vi "RT_cRIO_AIChar_v3.vi"() -> ()   [LabVIEW 2019]
uses:
  FPGA/TypeDefs/AO mode TabCtrl.ctl
  FPGA/TypeDefs/AI_channelEnum.ctl
  FPGA/TypeDefs/SamplingModeEnum.ctl
  <vilib>/NI/STM/SubVIs/MetaDataElement.ctl
  <vilib>/Platform/TimedLoop/XDataNode/timing_clust.ctl
  <vilib>/Platform/TimedLoop/XDataNode/nitl_modes.ctl
  <vilib>/Platform/TimedLoop/XDataNode/wakeup.ctl
  <vilib>/rvi/Analysis/host/Butterworth/config/Butterworth Filter Order.ctl
  <vilib>/rvi/Analysis/host/Butterworth/config/Butterworth Filter Type.ctl
  <vilib>/NI/STM/TCP/Write Meta Data (TCP Ref).vi
  <vilib>/NI/STM/TCP/Get Connection Reference (TCP).vi
  <vilib>/NI/STM/TCP/Write Meta Data (TCP Clst).vi
  <vilib>/FPGAPlugInAG/cRIO-9064/niLvFpga_Open_cRIO-9064.vi
  <vilib>/rvi/interface/common/dynamic/niFpgaDynamicAddResources.vi
  <vilib>/NI/STM/TCP/Write Message (TCP).vi
  <vilib>/rvi/Analysis/host/Private/Sample Rate To Loop Time (ticks).vi
  <vilib>/rvi/Analysis/host/Butterworth/config/BwScaledCoefficients.vi
  <vilib>/Utility/error.llb/Error Cluster From Error Code.vi
  <vilib>/rvi/errors/niLvFpgaAdjustHostInterfaceError.vi
  <vilib>/FPGAPlugInAG/Dynamic/niLvFpga_Close_Dynamic.vi
  <vilib>/rvi/interface/nirviOpenFPGA/nirviOpenFPGA.xnode
  FPGA Bitfiles/ainoisecharacter_FPGATarget2_FPGAcRIOMainv4_BvJefVyibFQ.lvbitx
  <vilib>/rvi/Analysis/host/Butterworth/XNode/ButterworthCoefficients.xnode
  <vilib>/rvi/interface/nirviReadWriteControl/nirviReadWriteControl.xnode
  <vilib>/Platform/TimedLoop/XDataNode/XDataNode.xnode
  <vilib>/rvi/interface/nirviCloseFPGA/nirviCloseFPGA.xnode
  <vilib>/Platform/TimedLoop/XDataNode/XDNodeRunTimeDep.lvlib
  Components/Timing/Timing.lvlib
  <vilib>/NI/STM/NI STM.lvlib
  <vilib>/rvi/interface/Simulation/niFpgaSimulationCallBeginRW.vi
  NiFpgaLv.dll
  <vilib>/rvi/Analysis/host/Public/NI_FpgaMspHost.lvlib
panel:
  in  "Sampling Mode":T1
  out "AI Process Freq.\ntoo high?":bool
  in  "AI Process Freq. [Hz]":dbl=20000.0 format="%#.3p"
  in  "Select Channel":T2=enum."AI1"
  in  "AO mode":T3=enum."100*AI"
  in  "AO Out [V]":fxp<+/-,18,5>
  in  "AI-chain LPF [Hz]":dbl=500.0 format="%#_6p"
  out "Sample Freq.\ntoo high?":bool
  in  "AO enable?":bool
  in  "Sample Freq [Hz]":dbl=300000.0 format="%#.3p"
  out "RT Loop Rate":dbl=5000.0 format="%.3p"
  out "# of iterations\n[STM write]":i32
  out "# elements \nFIFO buffer":u32
  out "Finished \nlate counter?":dbl
  in  "stop":bool
  # "- Open PC_SensorChar vi and run that VI as well to start capturing data!\n- Sampling Mode : \n     - LPF adds a  butterworth filter after the ADC conversion.\n     - 4pt. Avg adds a 4pt. Moving Avg before the LPF and after ADC."
  # "AO = \n100 * (AI value)"
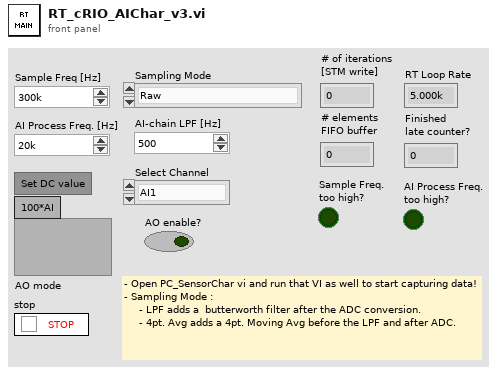
[diagram p1: front panel]
types:
  T1 = typedef "SamplingModeEnum.ctl" = enum16{"Raw", "M64 (ReSpl)", "M128 (ReSpl)", "M256 (ReSpl)", "MA (AI)", "4pt MA (AI) + M64 (ReSpl)", "LPF (Proc.)", "4pt MA (AI) + LPF (Proc.)", "4pt MA (Proc.) + LPF (Proc.)"}
  T2 = typedef "AI_channelEnum.ctl" = enum16{"AI0", "AI1", "AI2", "AI3"}
  T3 = typedef "AO mode TabCtrl.ctl" = enum32{"Set DC value", "100*AI"}
  T4 = typedef "NI STM.lvlib/MetaDataElement.ctl" = string
  T5 = typedef "NI STM.lvlib/TCP Connection Info.ctl" = cluster{"connection ID":refnum<k5>, "meta data":T4[]}
  T6 = typedef "XDNodeRunTimeDep.lvlib/timing_clust.ctl" = cluster{"Expected End [f-1]":u64, "Actual End [f-1]":u64, "Finished Late? [f-1]":bool, "Expected End [i-1]":u64, "Actual End [i-1]":u64, "Finished Late? [i-1]":bool, "Expected Start [i]":u64, "Actual Start [i]":u64, "Expected Start [f]":u64, "Actual Start [f]":u64, "Source Name":string, "Structure Name":string, "Period":i64, "Deadline":i64, "Offset":i64, "Start":i64, "Priority":i32, "Timeout":i32, "Mode":T7, "Wakeup Reason":T8, "Error":errorcluster, "Source Type":string, "Secondary Source Type":string, "Global End Time":u64, "Global Start Time":u64, "Frame Duration":u64, "Iteration Duration":u64, "Assigned CPU":i32, "I/O Scan Engine Mode":u32}
  T7 = typedef "XDNodeRunTimeDep.lvlib/nitl_modes.ctl" = enum32{"No Change", "Process missed periods, maintain original phase", "Discard missed periods, maintain original phase", "Process missed periods, ignore original phase", "Discard missed periods, ignore original phase"}
  T8 = typedef "XDNodeRunTimeDep.lvlib/wakeup.ctl" = enum32{"Normal", "Aborted", "Asynchronous wakeup", "Timing source error", "Timed loop error", "Timeout"}
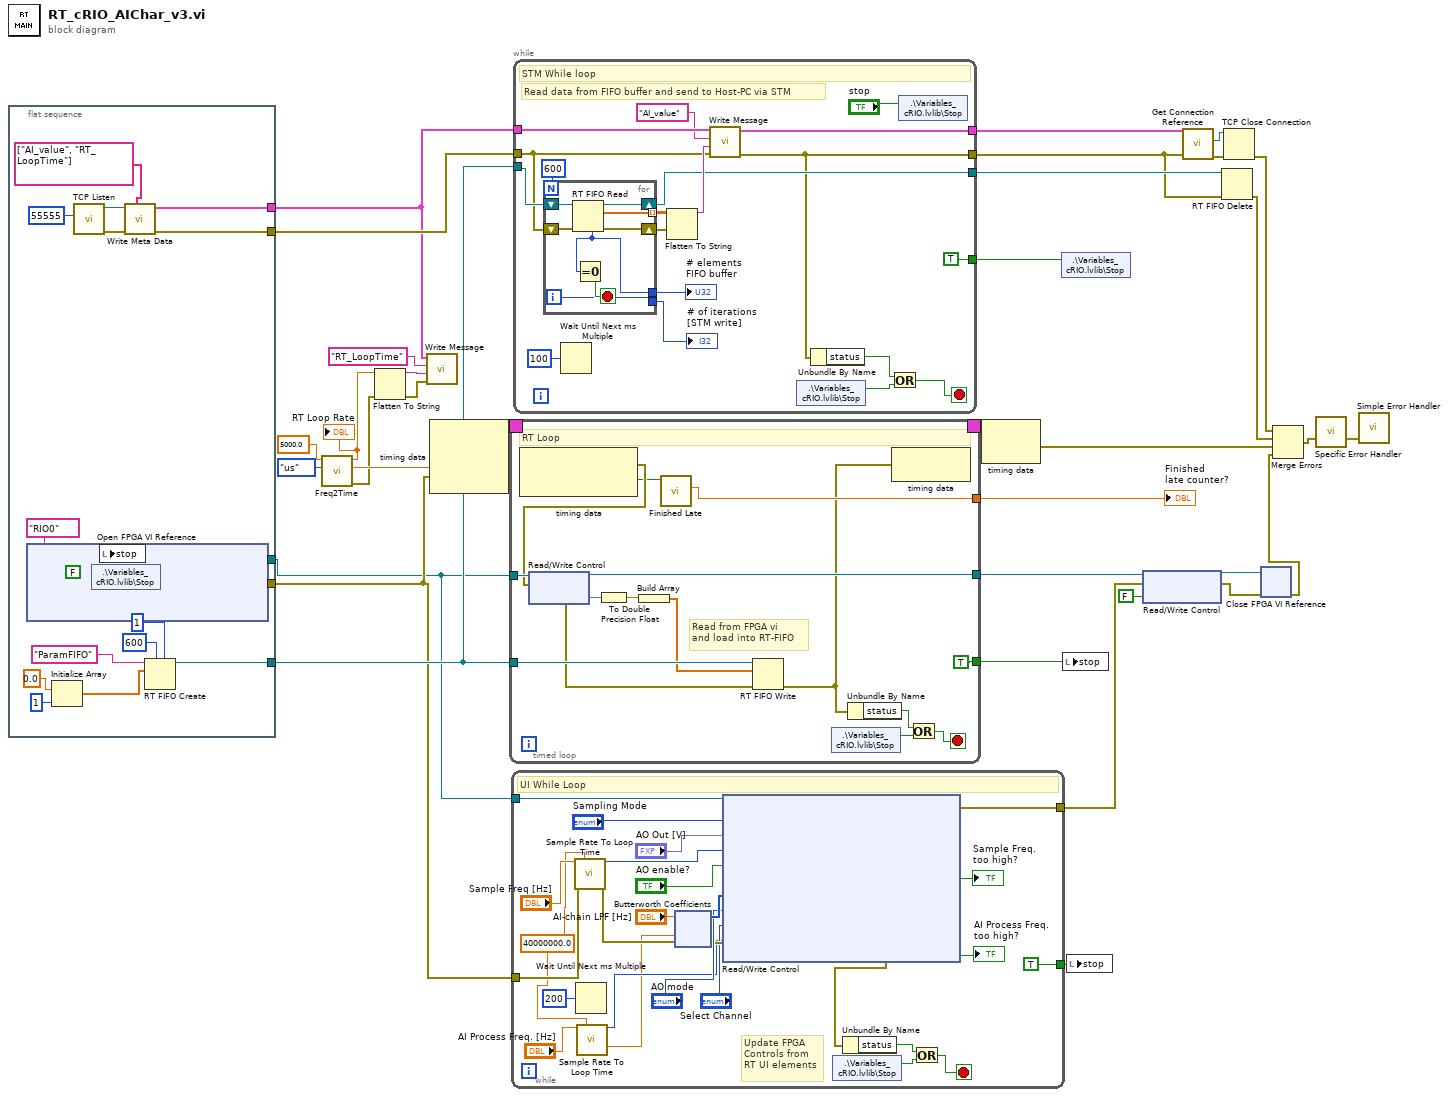
[diagram p0: block diagram]
diagram:
  n1 = flat-sequence {
    tunnel: [w51] -> w8
    tunnel: [w50] -> w7
    tunnel: [w45] -> w21
    tunnel: [w44] -> w29
    tunnel: [w43] -> w25
    frame #0 {
      w52 = FALSE ("Stop")
      n2 = xnode ("Open FPGA VI Reference")("resource name"=tag "RIO0") -> ("FPGA VI Reference Out"=w50:refnum<k20>, "error out"=w53:errorcluster)  [unwired: 1 in]
      n3 = Initialize Array(0.0 ("element"), 1 ("dimension size")) -> (w38:dbl[])
      n4 = call <vilib>:"TCP Listen.vi"("port"=u16 55555) -> ("error out"=w48:errorcluster, "connection ID"=w47:refnum<k5>)  [unwired: 6 in, 3 out]
      n5 = shared-variable ".\\Variables_cRIO.lvlib\\Stop"(w52, error in=w53) -> (error out=w51:errorcluster)
      n6 = local write "stop"(w52) -> ()
      n7 = call-poly <vilib>:"Write Meta Data.vi"("meta data"=T4[] ["AI_value", "RT_LoopTime"], "error in"=w48, "connection ID"=w47) -> ("error out"=w44:errorcluster, "connection info out"=w45:T5)  [unwired: 7 in]
      n8 = RT FIFO Create(0:"ParamFIFO" ("name (unnamed)"), 1:w38, 4:u32 600 ("size (10)"), 6:u32 1 ("elements in array (1)")) -> (8:w43:refnum<k33>)  [unwired: 4 in, 2 out]
    }
  }
  n9 = call "Freq2Time.vi"("Int. Time Unit"=enum16{"sec", "us", "ms"}."us", "Sample rate (Hz)"=5000.0 ("Period")) -> ("error out"=w15:errorcluster, "Int.  time [unit]"=w30:dbl, "New Sample rate (Hz)"=w17:dbl)  [unwired: 7 in]
  "RT Loop Rate" <- w17
  n10 = Flatten To String(anything=w17, error in (no error)=w15) -> (data string=w18:string, error out=w19:errorcluster)  [unwired: 2 in, 1 out]
  n11 = call-poly <vilib>:"Write Message.vi"("error in"=w19, "data"=w18, "name"="RT_LoopTime", "connection info in"=w21) -> ()  [unwired: 6 in, 2 out]
  n12 = node-c288(w30, w8) -> (w35:T6)  [unwired: 1 in]
  n13 = timed-loop {
    tunnel: w7 -> [w68]
    timing: w35 -> [_]
    timing-out: [_] -> w34
    tunnel: [w65] -> w33
    tunnel: w25 -> [w64]
    tunnel: [TRUE ("Stop")] -> w5
    tunnel: [w58] -> w6
    stop <- w57 stop-if-true
    # "Read from FPGA vi \nand load into RT-FIFO"
    # "RT Loop"
    n14 = node-c288() -> (w67:errorcluster, w66:bool)  [unwired: 1 in]
    n15 = xnode "Read/Write Control"("FPGA VI Reference In"=w68, "error in"=w67) -> ("FPGA VI Reference Out"=w58:refnum<k20>, "error out"=w59:errorcluster, "AI In [V]"=w63:fxp<+/-,25,5>)
    n16 = To Double Precision Float(number=w63) -> (double precision float=w62:dbl)
    n17 = Build Array(w62) -> (w61:dbl[])
    n18 = call "Finished Late.vi"("Finished \nLate?"=w66) -> ("# Finished\nLate counter"=w65:dbl)  [unwired: 8 in, 2 out]
    n19 = RT FIFO Write(0:w64, 1:w61, 3:w59) -> (11:w54:errorcluster)  [unwired: 2 in, 3 out]
    n20 = shared-variable ".\\Variables_cRIO.lvlib\\Stop"() -> (w56:bool)  [unwired: 1 in, 1 out]
    n21 = Unbundle By Name(w54) -> ("status"=w55:bool)
    n22 = node-c288(w54) -> ()  [unwired: 1 out]
    n23 = Or(x=w55, y=w56) -> (x .or. y?=w57:bool)
  }
  "Finished \nlate counter?" <- w33
  n24 = while {
    tunnel: w8 -> [w88]
    tunnel: w7 -> [w94]
    tunnel: [TRUE ("Stop")] -> w4
    tunnel: [w83] -> w3
    stop <- w85 stop-if-true
    w80 = 40000000.0 ("FPGA clock rate (Hz)")
    # "Update FPGA \nControls from\nRT UI elements"
    # "UI While Loop"
    n25 = call-poly <vilib>:"Sample Rate To Loop Time.vi"("sample rate (S/s)"="Sample Freq [Hz]", "FPGA clock rate (Hz)"=w80, "error in (no error)"=w88) -> ("count (ticks/S)"=w89:u32, "error out"=w87:errorcluster)  [unwired: 10 in, 1 out]
    n26 = Wait Until Next ms Multiple(millisecond multiple=u32 200) -> ()  [unwired: 1 out]
    n27 = call-poly <vilib>:"Sample Rate To Loop Time.vi"("sample rate (S/s)"="AI Process Freq. [Hz]", "FPGA clock rate (Hz)"=w80) -> ("count (ticks/S)"=w78:u32, "actual sample rate (S/s)"=w77:dbl)  [unwired: 11 in, 1 out]
    n28 = xnode "Butterworth Coefficients"("cutoff frequency (Hz)"="AI-chain LPF [Hz]", "sample rate (S/s)"=w77, "error in (no error)"=w87) -> ("scaled coefficients"=w97:i32[], "error out"=w82:errorcluster)
    n29 = xnode "Read/Write Control"("FPGA VI Reference In"=w94, "error in"=w82, "Sampling Mode"="Sampling Mode", "AO Out [V]"="AO Out [V]", "Sample Time [ticks]"=w89, "AO enable?"="AO enable?", "Scaled Butterworth Coeffs"=w97, "AO mode"="AO mode", "Select Channel"="Select Channel", "AI Process Time [ticks]"=w78) -> ("error out"=w83:errorcluster, "Unable to sample at desired Sample Rate?"=→"Sample Freq.\ntoo high?":bool, "AI Processing Loop Rate to high?"=→"AI Process Freq.\ntoo high?":bool)  [unwired: 1 out]
    n30 = shared-variable ".\\Variables_cRIO.lvlib\\Stop"() -> (w86:bool)  [unwired: 1 in, 1 out]
    n31 = Unbundle By Name(w83) -> ("status"=w84:bool)
    n32 = Or(x=w84, y=w86) -> (x .or. y?=w85:bool)
  }
  n33 = while {
    tunnel: w21 -> [w124]
    tunnel: w29 -> [w117]
    tunnel: [w122] -> w28
    tunnel: [w107] -> w23
    tunnel: w25 -> [w119]
    tunnel: [w116] -> w24
    tunnel: [TRUE ("Stop")] -> w1
    stop <- w109 stop-if-true
    # "Read data from FIFO buffer and send to Host-PC via STM"
    # "STM While loop"
    n34 = for {
      N: 600 -> [_]
      shift-right: [w130] -> w116
      shift-left: w119 -> [w133]
      shift-right: [w132] -> w118
      shift-left: w117 -> [w131]
      tunnel: [w129] -> w115
      tunnel: [w127] -> w114
      tunnel: [w126] -> w113 mode=indexing
      i -> [w127]
      stop <- w128 stop-if-true
      n35 = RT FIFO Read(0:w133, 3:w131) -> (7:w129:u32, 8:w130:refnum<k33>, 9:w126:dbl[], 11:w132:errorcluster)  [unwired: 2 in, 1 out]
      n36 = Equal To 0?(x=w129) -> (x = 0?=w128:bool)
    }
    "# elements \nFIFO buffer" <- w115
    "# of iterations\n[STM write]" <- w114
    n37 = Wait Until Next ms Multiple(millisecond multiple=u32 100) -> ()  [unwired: 1 out]
    n38 = Flatten To String(anything=w113, error in (no error)=w118) -> (data string=w121:string)  [unwired: 2 in, 2 out]
    n39 = call-poly <vilib>:"Write Message.vi"("error in"=w117, "data"=w121, "name"="AI_value", "connection info in"=w124) -> ("error out"=w107:errorcluster, "connection info out"=w122:T5)  [unwired: 6 in]
    n40 = shared-variable ".\\Variables_cRIO.lvlib\\Stop"() -> (w110:bool)  [unwired: 1 in, 1 out]
    n41 = Unbundle By Name(w107) -> ("status"=w108:bool)
    n42 = Or(x=w108, y=w110) -> (x .or. y?=w109:bool)
    n43 = shared-variable ".\\Variables_cRIO.lvlib\\Stop"("stop") -> ()  [unwired: 1 in, 1 out]
  }
  n44 = node-c288(w34) -> (w16:errorcluster)
  n45 = shared-variable ".\\Variables_cRIO.lvlib\\Stop"(w1) -> ()  [unwired: 1 in, 1 out]
  n46 = local write "stop"(w5) -> ()
  n47 = local write "stop"(w4) -> ()
  n48 = xnode "Read/Write Control"("FPGA VI Reference In"=w6, "error in"=w3, "AO enable?"=FALSE ("AO enabled?")) -> ("FPGA VI Reference Out"=w11:refnum<k20>, "error out"=w10:errorcluster)
  n49 = call-poly <vilib>:"Get Connection Reference.vi"("error in"=w23, "connection info in"=w28) -> ("error out"=w27:errorcluster, "connection ID out"=w26:refnum<k5>)  [unwired: 7 in, 1 out]
  n50 = RT FIFO Delete(0:w24, 3:w23) -> (11:w22:errorcluster)  [unwired: 1 in]
  n51 = TCP Close Connection(connection ID=w26, error in (no error)=w27) -> (error out=w12:errorcluster)  [unwired: 1 in, 1 out]
  n52 = xnode "Close FPGA VI Reference"("FPGA VI Reference In"=w11, "error in"=w10) -> ("error out"=w2:errorcluster)
  n53 = Merge Errors(w12, w22, w16, w2) -> (w14:errorcluster)
  n54 = call "Specific Error Handler"("Error to Check"=w14) -> ("error out"=w13:errorcluster)  [unwired: 11 in, 3 out]
  n55 = call <vilib>:"Simple Error Handler.vi"("error in (no error)"=w13) -> ()  [unwired: 4 in, 5 out]
